vi "IsotonicRegression.vi"(8 "error in":errorcluster) -> (0 "error out":errorcluster, 3 "out":refnum<class "IsotonicRegression.lvclass">)   [LabVIEW 2020]
doc: "Isotonic regression model.\n\n Read more in the :ref:`User Guide <isotonic>`.\n\n .. versionadded:: 0.13\n\n Parameters\n ----------\n y_min : float, default=None\n Lower bound on the lowest predicted value (the minimum value may\n still be higher). If not set, defaults to -inf.\n\n y_max : float, default=None\n Upper bound on the highest predicted value (the maximum may still be\n lower). If not set, defaults to +inf.\n\n increasing : bool or 'auto', default=True\n Determines whether the predictions should be constrained to increase\n or decrease with `X`. 'auto' will decide based on the Spearman\n correlation estimate's sign.\n\n out_of_bounds : {'nan', 'clip', 'raise'}, default='nan'\n Handles how `X` values outside of the training domain are handled\n during prediction.\n\n - 'nan', predictions will be NaN.\n - 'clip', predictions will be set to the value corresponding to\n the nearest train interval endpoint.\n - 'raise', a `ValueError` is raised.\n\n Attributes\n ----------\n X_min_ : float\n Minimum value of input array `X_` for left bound.\n\n X_max_ : float\n Maximum value of input array `X_` for right bound.\n\n X_thresholds_ : ndarray of shape (n_thresholds,)\n Unique ascending `X` values used to interpolate\n the y = f(X) monotonic function.\n\n .. versionadded:: 0.24\n\n y_thresholds_ : ndarray of shape (n_thresholds,)\n De-duplicated `y` values suitable to interpolate the y = f(X)\n monotonic function.\n\n .. versionadded:: 0.24\n\n f_ : function\n The stepwise interpolating function that covers the input domain ``X``.\n\n increasing_ : bool\n Inferred value for ``increasing``.\n\n Notes\n -----\n Ties are broken using the secondary method from de Leeuw, 1977.\n\n References\n ----------\n Isotonic Median Regression: A Linear Programming Approach\n Nilotpal Chakravarti\n Mathematics of Operations Research\n Vol. 14, No. 2 (May, 1989), pp. 303-308\n\n Isotone Optimization in R : Pool-Adjacent-Violators\n Algorithm (PAVA) and Active Set Methods\n de Leeuw, Hornik, Mair\n Journal of Statistical Software 2009\n\n Correctness of Kruskal's algorithms for monotone regression with ties\n de Leeuw, Psychometrica, 1977\n\n \nAvailable methods:\nGet Attributes\nGet Params\nSet Params"
uses:
  IsotonicRegression/IsotonicRegression.lvclass
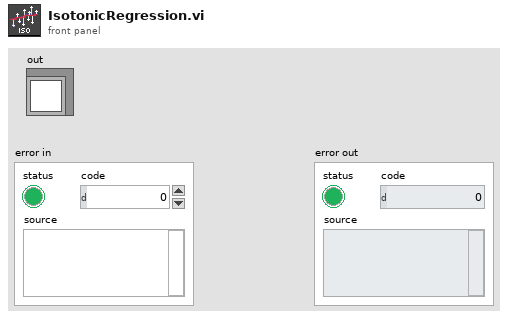
[diagram p1: front panel]
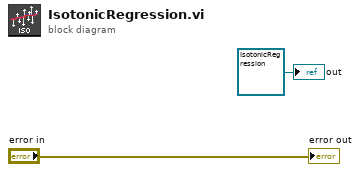
[diagram p0: block diagram]
diagram:
  "out" <- refnum<class "IsotonicRegression.lvclass"> refnum ("model")
  "error out" <- "error in"
